vi "txtArr to Excel.vi"(5 "ResultArrayIn":string[](array[string]), 7 "TestStage":string, 9 "SN":string, 11 "error in (no error)":errorcluster) -> (8 "MagResult":string[](array[string]), 15 "error out":errorcluster)   [LabVIEW 2017]
uses:
  <vilib>/addons/_office/excel.llb/Excel Easy Table (str).vi
  <vilib>/addons/_office/excel.llb/Excel Get Data (str).vi
  <vilib>/Utility/NIReport.llb/NI_report.lvclass
  <vilib>/addons/_office/NI_ReportGenerationToolkit.lvlib
  <vilib>/Utility/NIReport.llb/Excel/NI_Excel.lvclass
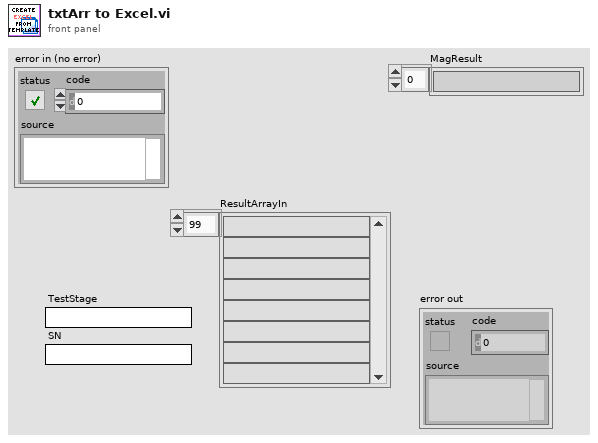
[diagram p1: front panel]
types:
  T1 = enum16{"maximized", "minimized", "normal", "no change"}
  T2 = enum16{"Standard Report", "HTML", "Word", "Excel"}
  T3 = enum16{"open", "replace", "create", "open or create", "replace or create", "replace or create with confirmation"}
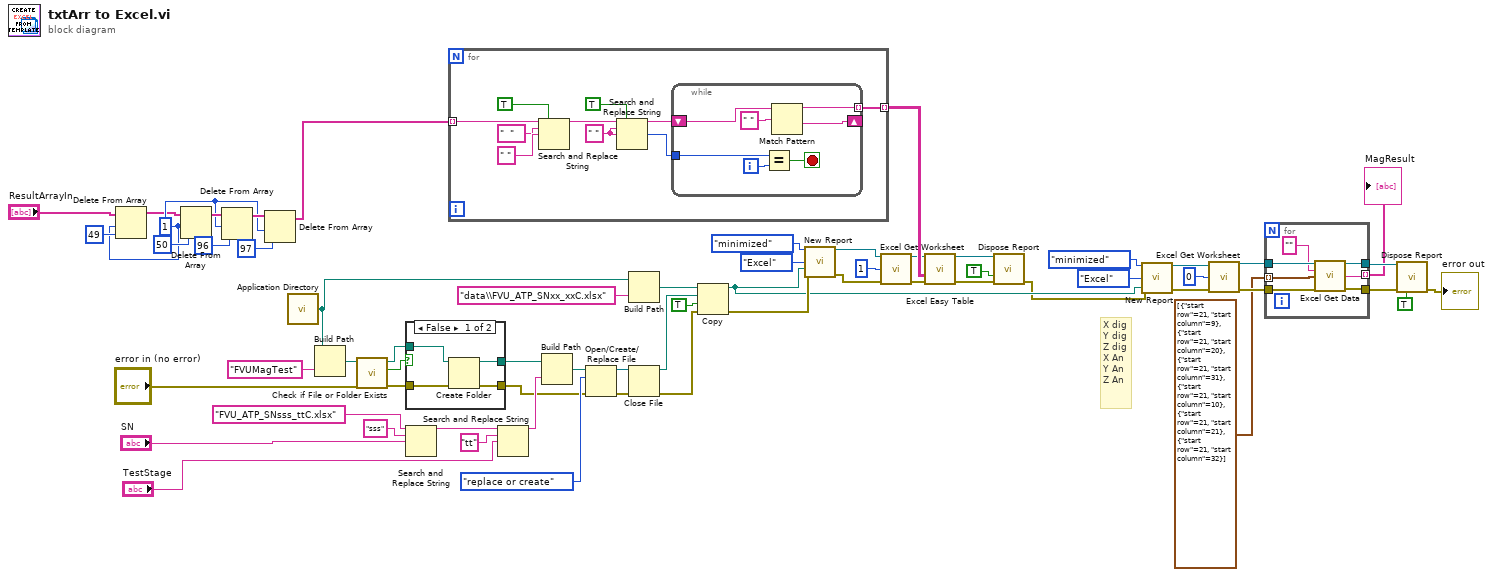
[diagram p0: block diagram]
diagram:
  w3 = 1 ("length")
  # "X dig\nY dig\nZ dig\nX An\nY An\nZ An"
  n1 = Delete From Array(array="ResultArrayIn", length=w3, index=49) -> (array with subset deleted=w1:string[])  [unwired: 1 out]
  n2 = Delete From Array(array=w1, length=w3, index=50) -> (array with subset deleted=w9:string[])  [unwired: 1 out]
  n3 = Delete From Array(array=w9, length=w3, index=96) -> (array with subset deleted=w5:string[])  [unwired: 1 out]
  n4 = Delete From Array(array=w5, length=w3, index=97) -> (array with subset deleted=w4:string[])  [unwired: 1 out]
  n5 = call <vilib>:"Application Directory.vi"() -> ("Application Directory"=w30:path)
  n6 = Build Path(base path=w30, name or relative path="FVUMagTest") -> (appended path=w37:path)
  n7 = call <vilib>:"Check if File or Folder Exists.vi"("error in (no error)"="error in (no error)", "path"=w37) -> ("error out"=w39:errorcluster, "file or folder exists?"=w36:bool, "dup path"=w38:path)  [unwired: 7 in]
  n8 = case shown="False" w36 {
    tunnel: w39 -> [w66 w67]
    tunnel: w38 -> [w65 w68]
    tunnel: [w64 w68] -> w33
    tunnel: [w63 w67] -> w28
    frame False {
      n9 = Create Folder(path (use dialog)=w65, error in=w66) -> (created path=w64:path, error out=w63:errorcluster)  [unwired: 1 in, 1 out]
    }
    frame True {
    }
  }
  n10 = Search and Replace String(input string="FVU_ATP_SNsss_ttC.xlsx" ("name or relative path"), search string="sss", replace string="SN") -> (result string=w43:string)  [unwired: 5 in, 3 out]
  n11 = for {
    tunnel: w4 -> [w72] mode=indexing
    tunnel: [w75] -> w60 mode=indexing
    w76 = " " ("regular expression")
    n12 = Search and Replace String(replace all?=TRUE ("replace all? (F)"), input string=w72, search string="  " ("regular expression"), replace string=" " ("regular expression")) -> (result string=w71:string)  [unwired: 4 in, 3 out]
    n13 = Search and Replace String(replace all?=TRUE ("replace all? (F)"), input string=w71, search string=w76, replace string=w76) -> (result string=w69:string, number of replacements=w77:i32)  [unwired: 4 in, 2 out]
    n14 = while {
      shift-right: [w83] -> _
      shift-left: w69 -> [w85]
      tunnel: [w82] -> w75 mode=indexing
      tunnel: w77 -> [w81]
      i -> [w79]
      stop <- w80 stop-if-true
      n15 = Equal?(x=w81, y=w79) -> (x = y?=w80:bool)
      n16 = Match Pattern(string=w85, regular expression=" ") -> (before substring=w82:string, after substring=w83:string)  [unwired: 1 in, 2 out]
    }
  }
  n17 = Search and Replace String(input string=w43, search string="tt", replace string="TestStage") -> (result string=w34:string)  [unwired: 5 in, 3 out]
  n18 = Build Path(base path=w33, name or relative path=w34) -> (appended path=w31:path)
  n19 = Open/Create/Replace File(file path (use dialog)=w31, error in=w28, operation (0:open)=T3."replace or create") -> (refnum out=w47:refnum<file>, error out=w48:errorcluster)  [unwired: 3 in, 1 out]
  n20 = Build Path(base path=w30, name or relative path="data\\FVU_ATP_SNxx_xxC.xlsx") -> (appended path=w50:path)
  n21 = Close File(refnum=w47, error in=w48) -> (path=w46:path, error out=w27:errorcluster)
  n22 = Copy(8:w27, 9:TRUE ("overwrite (F)"), 10:w46, 11:w50) -> (0:w26:errorcluster, 3:w20:path)  [unwired: 1 in, 1 out]
  n23 = call <vilib>:"New Report.vi"("window state (normal)"=T1."minimized", "report type"=T2."Excel", "template (empty)"=w20, "error in (no error)"=w26) -> ("report out"=w59:refnum<class "NI_report.lvclass">, "error out"=w58:errorcluster)  [unwired: 10 in]
  n24 = call <vilib>:"Excel Get Worksheet.vi"("report in"=w59, "worksheet index (0)"=1, "error in (no error)"=w58) -> ("report out"=w57:refnum<class "NI_report.lvclass">, "error out"=w56:errorcluster)  [unwired: 11 in]
  n25 = call-poly <vilib>:"Excel Easy Table.vi"("report in"=w57, "text data"=w60, "error in (no error)"=w56) -> ("report out"=w53:refnum<class "NI_report.lvclass">, "error out"=w52:errorcluster)  [unwired: 8 in, 3 out]
  n26 = call-dynamic "Dispose Report.vi"("report in"=w53, "save changes? (F)"=TRUE, "error in (no error)"=w52) -> ("error out"=w19:errorcluster)  [unwired: 12 in]
  n27 = call <vilib>:"New Report.vi"("window state (normal)"=T1."minimized", "report type"=T2."Excel", "template (empty)"=w20, "error in (no error)"=w19) -> ("report out"=w22:refnum<class "NI_report.lvclass">, "error out"=w23:errorcluster)  [unwired: 10 in]
  n28 = call <vilib>:"Excel Get Worksheet.vi"("report in"=w22, "worksheet index (0)"=0, "error in (no error)"=w23) -> ("report out"=w17:refnum<class "NI_report.lvclass">, "error out"=w18:errorcluster)  [unwired: 11 in]
  n29 = for {
    tunnel: w18 -> [w92]
    tunnel: w17 -> [w91]
    tunnel: cluster{"start row":i32, "start column":i32}[] [{"start row"=21, "start column"=9}, {"start row"=21, "start column"=20}, {"start row"=21, "start column"=31}, {"start row"=21, "start column"=10}, {"start row"=21, "start column"=21}, {"start row"=21, "start column"=32}] -> [w89] mode=indexing
    tunnel: [w88] -> w13
    tunnel: [w87] -> w12
    tunnel: [w86] -> w11 mode=indexing
    n30 = call-poly <vilib>:"Excel Get Data.vi"("report in"=w91, "data type"="", "start (0, 0)"=w89, "error in (no error)"=w92) -> ("report out"=w88:refnum<class "NI_report.lvclass">, "data"=w86:string, "error out"=w87:errorcluster)  [unwired: 9 in]
  }
  "MagResult" <- w11
  n31 = call-dynamic "Dispose Report.vi"("report in"=w13, "error in (no error)"=w12, "close report? (T)"=TRUE) -> ("error out"=→"error out":errorcluster)  [unwired: 12 in]
